vi "Test - Thermal Chamber Controller_DQMH - Update Heater State 1-test_harness.vi"(11 "test case ID":string) -> (3 "result":bool)   [LabVIEW 2018]
uses:
  Libraries/Thermal Chamber Controller_DQMH/Thermal Chamber Controller_DQMH.lvlib
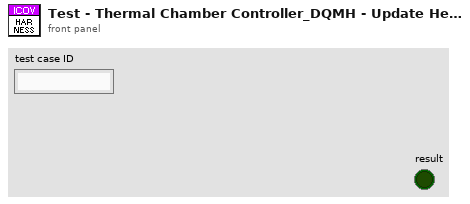
[diagram p1: front panel]
types:
  T1 = typedef "Thermal Chamber Controller_DQMH.lvlib/Heater State--enum.ctl" = enum16{"Heater Enabled", "Heater Disabled"}
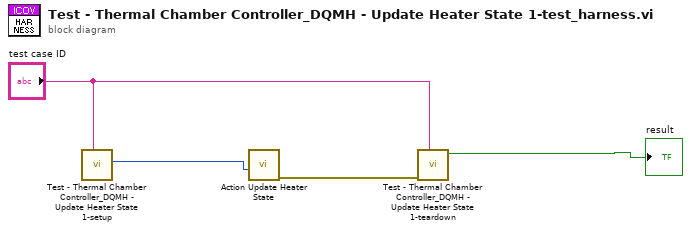
[diagram p0: block diagram]
diagram:
  n1 = call "Test - Thermal Chamber Controller_DQMH - Update Heater State 1-setup.vi"("test case ID"="test case ID") -> ("Heater State"=w3:T1)  [unwired: 10 in]
  n2 = call "Action Update Heater State.vi"("Heater State"=w3) -> ("error out"=w2:errorcluster)  [unwired: 10 in]
  n3 = call "Test - Thermal Chamber Controller_DQMH - Update Heater State 1-teardown.vi"("test case ID"="test case ID", "error in (no error)"=w2) -> ("result"=→"result":bool)  [unwired: 9 in]
